vi "Main.vi"() -> ()   [LabVIEW 2023, in "VeriStand Console.lvlib"]
uses:
  VeriStand Console.lvlib
  Message.ctl
  SM Data.ctl
  <vilib>/net/SSH/Client/OpenSSH/OpenSSH Client.lvclass
  Message Queue.ctl
  Login Info.ctl
  <vilib>/net/SSH/NI_SSH.lvlib
panel:
  in  "Disconnect":bool
  out "Connected?":bool
  in  "Connect":bool
  in  "Password":string
  in  "Username":string
  in  "Target Address":string
  in  "Stop":bool
  in  "UI Settings":bool
  out "Console":string
  out "return code":i32
  out "standard error":string
  out "SM Debug Data":T1
  out "elements":T2[](array[typedef])
  out "# elements in queue":i32
  out "Poll rate (s)":dbl
  # "Debug"
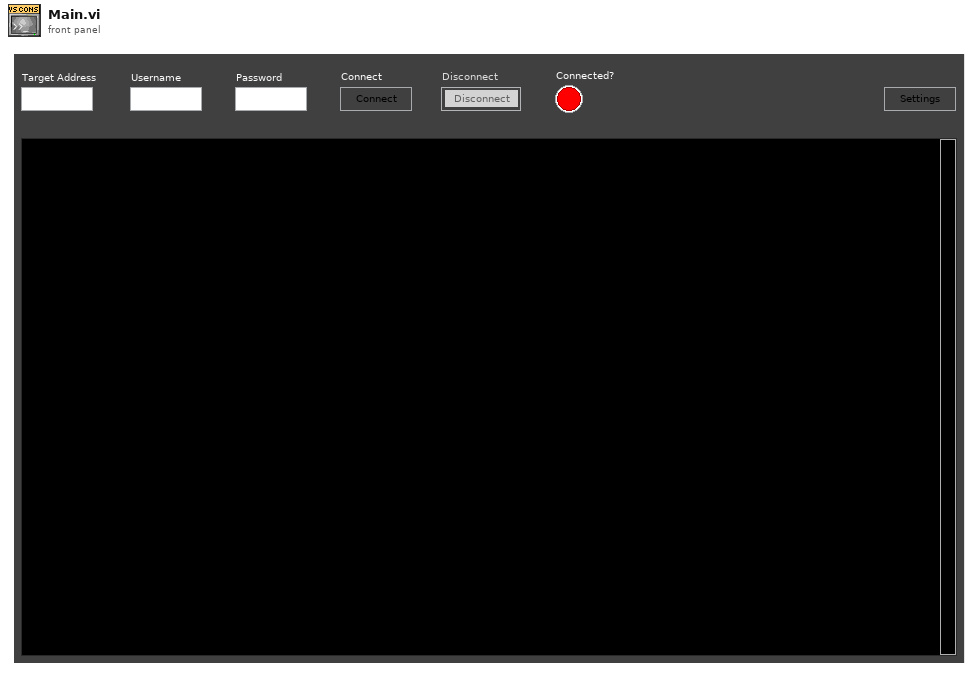
[diagram p1: front panel]
types:
  T1 = typedef "VeriStand Console.lvlib/SM Data.ctl" = cluster{"Connected?":bool, "User@host":string, "NI_SSH.lvlib:OpenSSH Client":refnum<class "OpenSSH Client.lvclass">, "Log file name":string, "Current text":string, "Scroll To Bottom?":bool}
  T2 = typedef "VeriStand Console.lvlib/Message.ctl" = cluster{"Message":string, "Message Data":variant}
  T3 = typedef "VeriStand Console.lvlib/Message Queue.ctl" = refnum<queue>
  T4 = enum8{"Enabled", "Disabled", "Disabled and Grayed Out"}
  T5 = typedef "VeriStand Console.lvlib/Login Info.ctl" = cluster{"Target IP Address":string, "Username":string, "Password":string, "Flush?":bool}
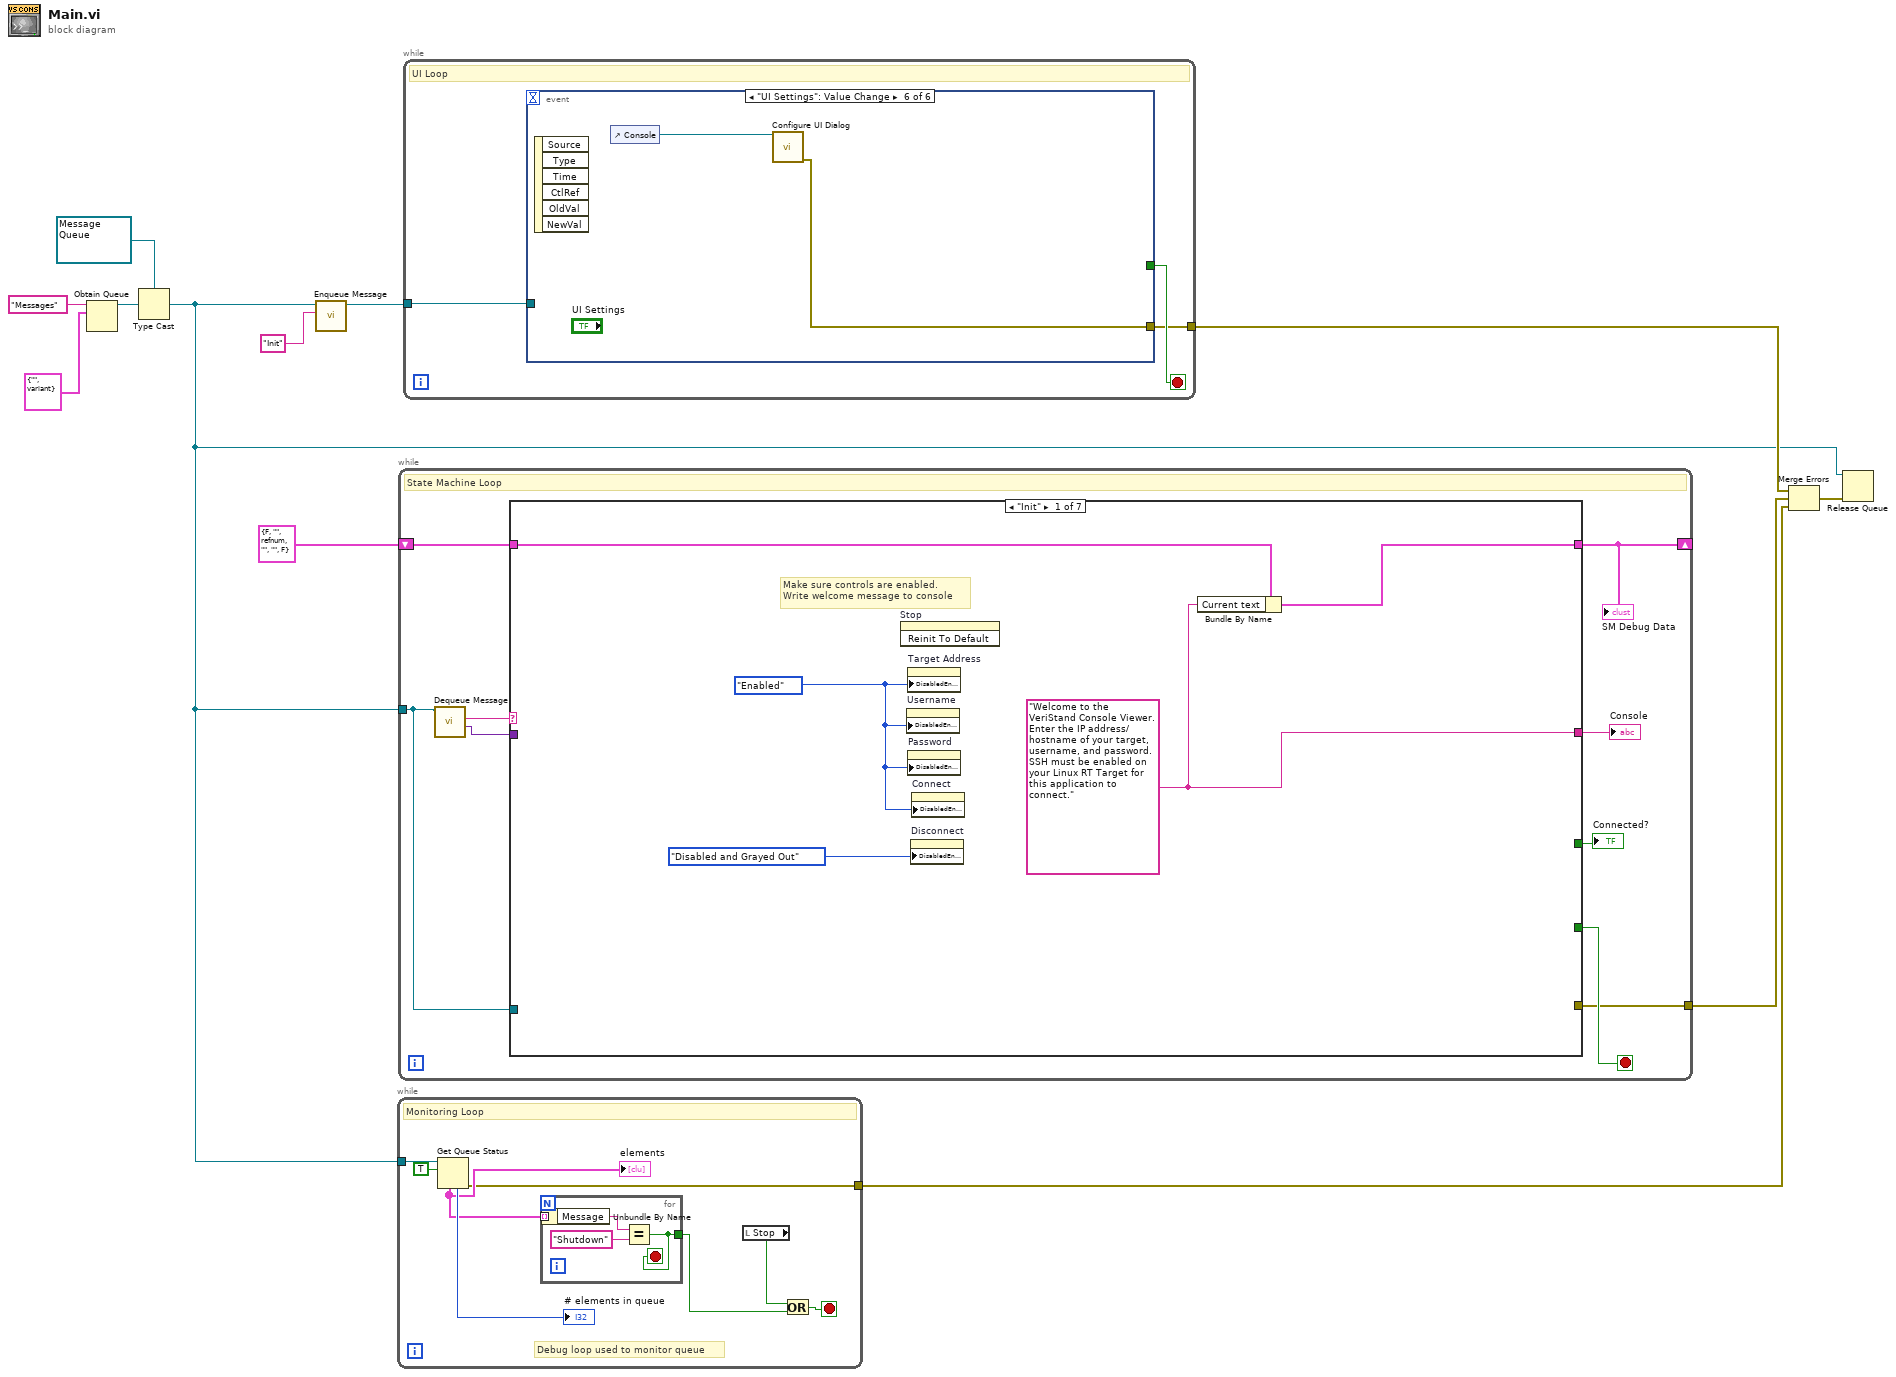
[diagram p0: block diagram]
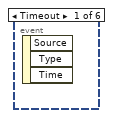
[diagram p2: hidden frame]
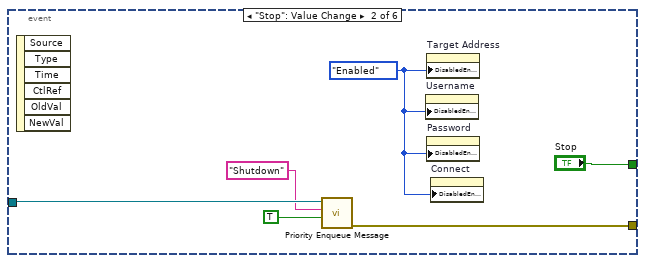
[diagram p3: hidden frame]
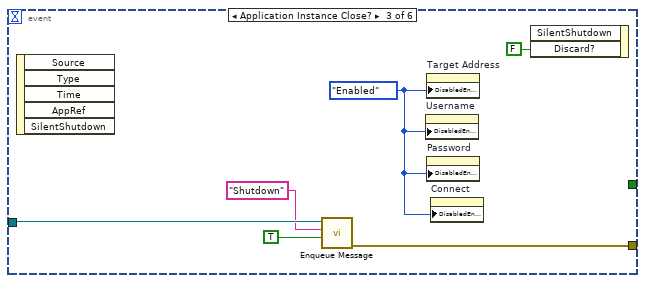
[diagram p4: hidden frame]
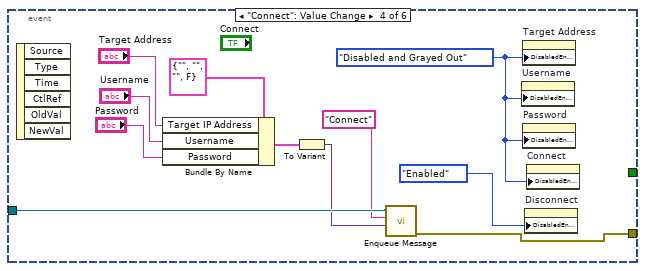
[diagram p5: hidden frame]
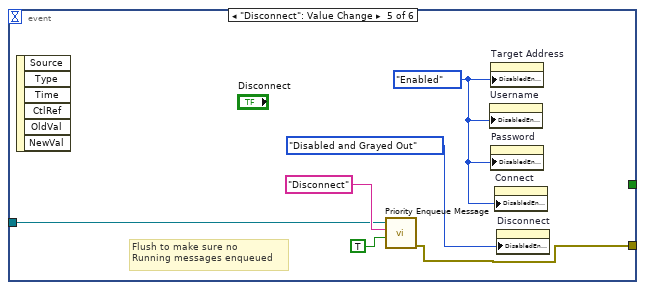
[diagram p6: hidden frame]
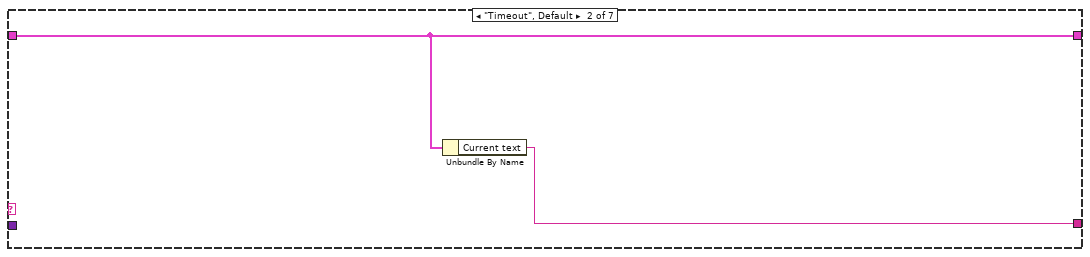
[diagram p7: hidden frame]
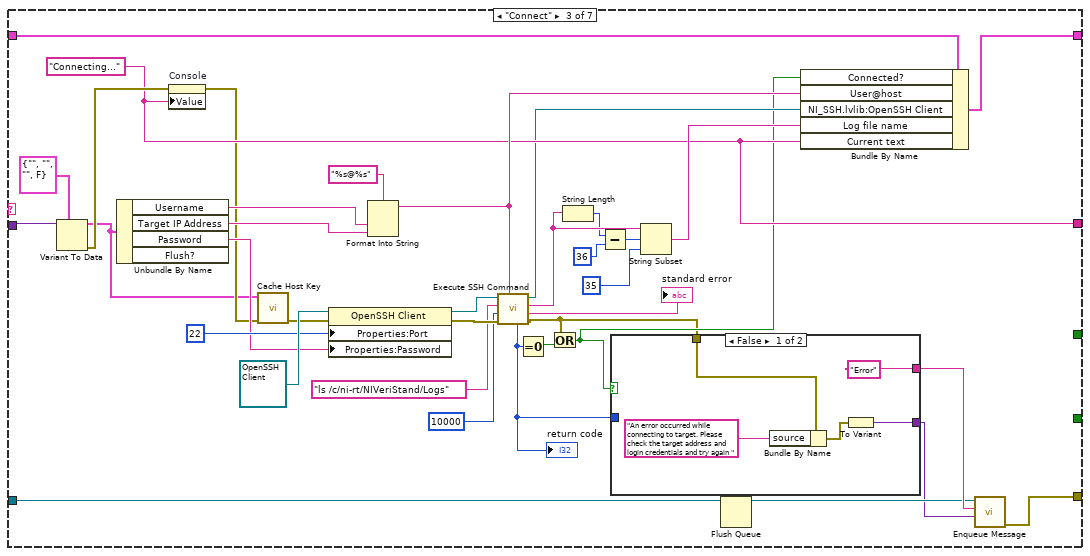
[diagram p8: hidden frame]
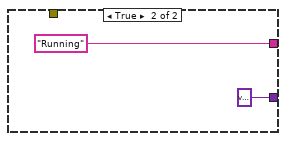
[diagram p9: hidden frame]
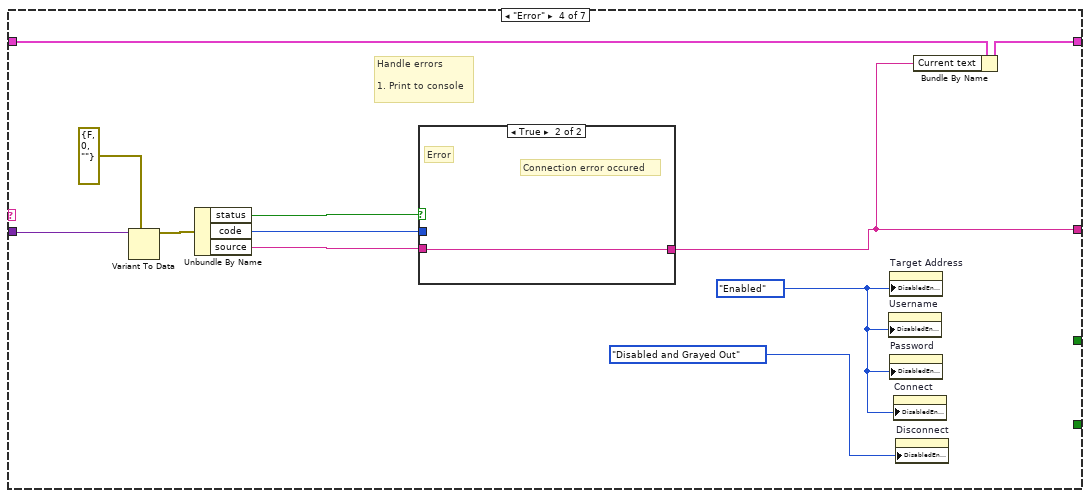
[diagram p10: hidden frame]
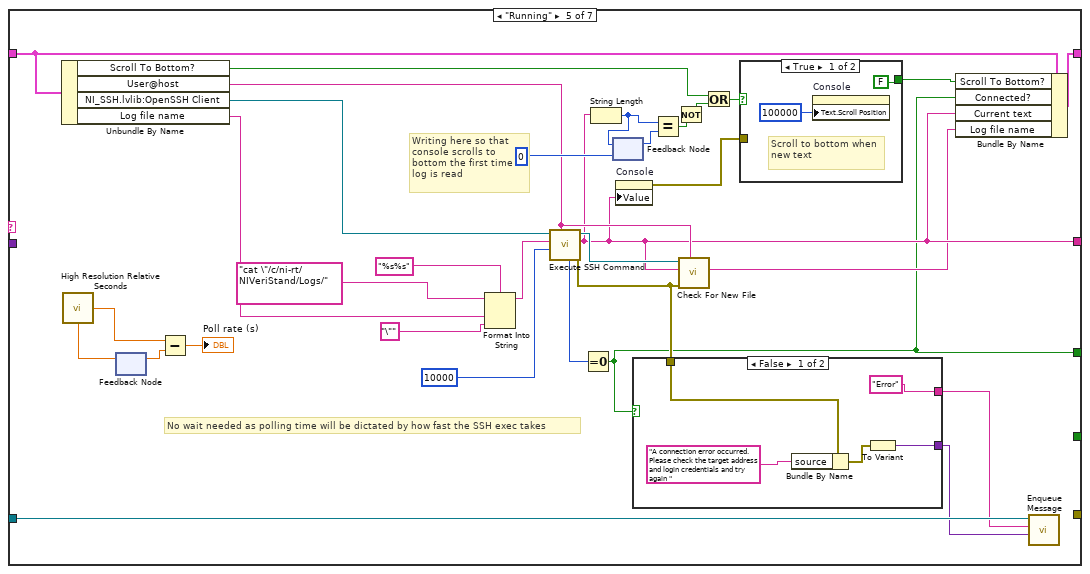
[diagram p12: hidden frame]
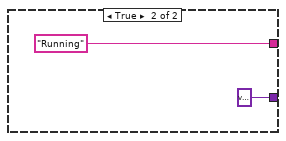
[diagram p13: hidden frame]
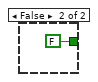
[diagram p14: hidden frame]
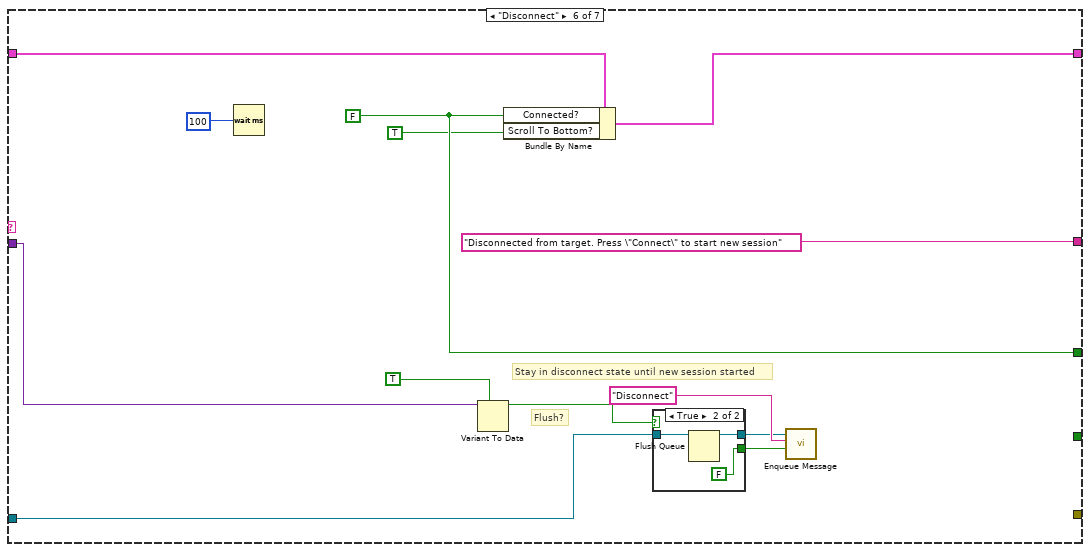
[diagram p15: hidden frame]
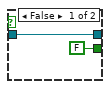
[diagram p16: hidden frame]
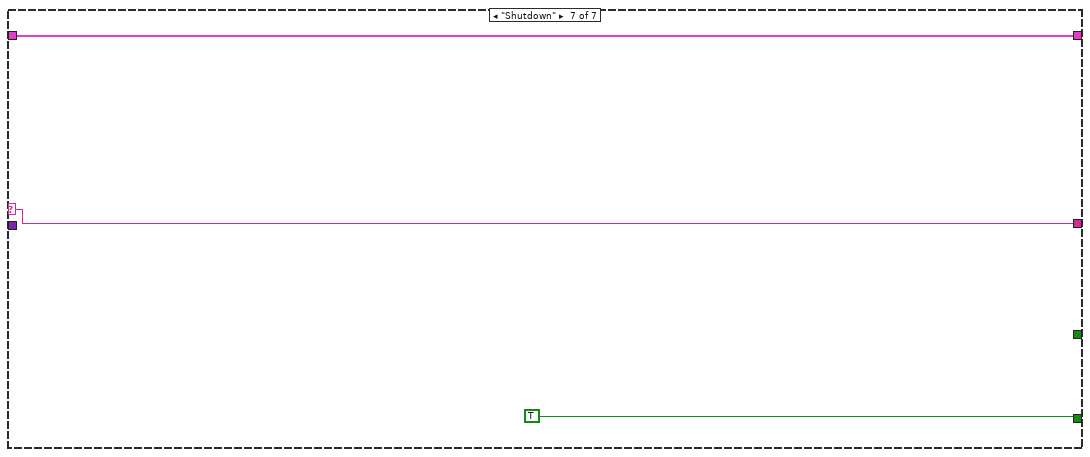
[diagram p17: hidden frame]
diagram:
  n1 = Obtain Queue(name (unnamed)="Messages", element data type=T2 {"Message"="", "Message Data"=variant} ("Message")) -> (queue out=w10:refnum<queue>)  [unwired: 3 in, 2 out]
  n2 = Type Cast(type=T3 refnum ("queue out"), x=w10) -> (*(type *) &x=w1:T3)
  n3 = call "Enqueue Message.vi"("Queue In"=w1, "Message"="Init") -> ("Queue Out"=w6:T3)  [unwired: 6 in, 1 out]
  n4 = while {
    tunnel: w1 -> [w20]
    tunnel: [w16] -> w4
    stop <- w15 stop-if-true
    # "Debug loop used to monitor queue"
    # "Monitoring Loop"
    n5 = Get Queue Status(queue=w20, return elements? (F)=TRUE) -> (error out=w16:errorcluster, # elements in queue=→"# elements in queue":i32, elements=w18:T2[])  [unwired: 1 in, 5 out]
    "elements" <- w18
    n6 = for {
      tunnel: w18 -> [w24] mode=indexing
      tunnel: [w21] -> w14
      stop <- w21 stop-if-true
      n7 = Unbundle By Name(w24) -> ("Message"=w23:string)
      n8 = Equal?(x=w23, y="Shutdown") -> (x = y?=w21:bool)
    }
    n9 = local read "Stop"() -> (w13:bool)
    n10 = Or(x=w13, y=w14) -> (x .or. y?=w15:bool)
  }
  n11 = while {
    tunnel: w1 -> [w26]
    shift-right: [w27] -> _
    shift-left: T1 {"Connected?"=FALSE, "User@host"="", "NI_SSH.lvlib:OpenSSH Client"=refnum, "Log file name"="", "Current text"="", "Scroll To Bottom?"=FALSE} ("SM Data") -> [w28]
    tunnel: [w25] -> w3
    stop <- w33 stop-if-true
    # "State Machine Loop"
    n12 = call "Dequeue Message.vi"("Queue In"=w26) -> ("Message Data"=w31:variant, "Message"=w32:string)  [unwired: 6 in, 3 out]
    n13 = case shown="\"Init\"" w32 {
      selector: w32 -> [_ _ _ _ _ _ w158]
      tunnel: [w35 w40 w52 w87 w104 "Disconnected from target. Press \"Connect\" to start new session" ("standard output") w158] -> w30
      tunnel: [_ _ _ _ _ _ TRUE] -> w33
      tunnel: w31 -> [_ _ w77 w94 _ w143 _]
      tunnel: [_ _ _ _ w98 w148 _] -> w29
      tunnel: w28 -> [w37 w39 w64 w95 w110 w151 w157]
      tunnel: [w36 w39 w63 w88 w109 w150 w157] -> w27
      tunnel: w26 -> [_ _ w55 _ w122 w144 _]
      tunnel: [_ _ w54 _ _ _ _] -> w25
      frame "Init" {
        w38 = T4."Enabled" ("Disabled")
        w35 = "Welcome to the VeriStand Console Viewer. Enter the IP address/hostname of your target, username, and password. SSH must be enabled on your Linux RT Target for this application to connect." ("standard output")
        # "Make sure controls are enabled. \nWrite welcome message to console"
        n14 = invoke on="Stop" class="Bool (strict)" method="Reinit To Default"() -> ()  [unwired: 3 in, 3 out]
        n15 = property on="Username" class="Str"("DisabledEnum"=w38) -> ()  [unwired: 2 in, 2 out]
        n16 = property on="Target Address" class="Str"("DisabledEnum"=w38) -> ()  [unwired: 2 in, 2 out]
        n17 = property on="Password" class="Str"("DisabledEnum"=w38) -> ()  [unwired: 2 in, 2 out]
        n18 = property on="Disconnect" class="Bool"("DisabledEnum"=T4."Disabled and Grayed Out" ("Disabled")) -> ()  [unwired: 2 in, 2 out]
        n19 = property on="Connect" class="Bool"("DisabledEnum"=w38) -> ()  [unwired: 2 in, 2 out]
        n20 = Bundle By Name(cluster=w37, "Current text"=w35) -> (w36:T1)
      }
      frame "Timeout", Default {
        n21 = Unbundle By Name(w39) -> ("Current text"=w40:string)
      }
      frame "Connect" {
        w52 = "Connecting..." ("standard output")
        n22 = Variant To Data(type=T5 {"Target IP Address"="", "Username"="", "Password"="", "Flush?"=FALSE} ("Login Info"), Variant=w77) -> (data=w44:T5, error out=w53:errorcluster)  [unwired: 1 in]
        n23 = Unbundle By Name(w44) -> ("Username"=w71:string, "Target IP Address"=w70:string, "Password"=w68:string)  [unwired: 1 out]
        n24 = property on="Console" class="Str"(error in=w53, "Value"=w52) -> (error out=w45:errorcluster)  [unwired: 1 in, 1 out]
        n25 = call "Cache Host Key.vi"("error in (no error)"=w45, "Login Info"=w44) -> ("error out"=w46:errorcluster)  [unwired: 9 in]
        n26 = property class="OpenSSH Client"(reference=refnum<class "OpenSSH Client.lvclass"> refnum ("NI_SSH.lvlib:OpenSSH Client"), error in=w46, "Properties:Port"=u16 22 ("Port"), "Properties:Password"=w68) -> (reference out=w74:refnum<class "OpenSSH Client.lvclass">, error out=w73:errorcluster)
        n27 = Format Into String(format string="%s@%s", w71, w70) -> (resulting string=w66:string)  [unwired: 2 in, 1 out]
        n28 = call <vilib>:"Execute SSH Command.vi"("user@host"=w66, "error in (no error)"=w73, "timeout (ms)"=10000, "command line"="ls /c/ni-rt/NIVeriStand/Logs", "session in"=w74) -> ("error out"=w41:errorcluster, "standard error"=→"standard error":string, "standard output"=w62:string, "session out"=w48:refnum<class "OpenSSH Client.lvclass">, "return code"=w49:i32)  [unwired: 2 in]
        "return code" <- w49
        n29 = Equal To 0?(x=w49) -> (x = 0?=w42:bool)
        n30 = Or(x=w41, y=w42) -> (x .or. y?=w43:bool)
        n31 = String Length(string=w62) -> (length=w60:i32)
        n32 = Subtract(x=w60, y=36) -> (x-y=w61:i32)
        n33 = case shown="False" w43 {
          tunnel: ["Error" ("Message") "Running" ("Message")] -> w65
          tunnel: [w80 variant ("Variant")] -> w51
          tunnel: w49 -> [_ _]
          tunnel: w41 -> [w78 _]
          frame False {
            n34 = Bundle By Name(cluster=w78, "source"="An error occurred while connecting to target. Please check the target address and login credentials and try again " ("Message")) -> (w81:errorcluster)
            n35 = To Variant(anything=w81) -> (Variant=w80:variant)
          }
          frame True {
          }
        }
        n36 = String Subset(string=w62, offset (0)=w61, length (rest)=35 ("length (rest)")) -> (substring=w58:string)
        n37 = Flush Queue(queue=w55) -> (queue out=w56:T3)  [unwired: 1 in, 2 out]
        n38 = Bundle By Name(cluster=w64, "Connected?"=w43, "User@host"=w66, "NI_SSH.lvlib:OpenSSH Client"=w48, "Log file name"=w58, "Current text"=w52) -> (w63:T1)
        n39 = call "Enqueue Message.vi"("Queue In"=w56, "Message"=w65, "Message Data"=w51) -> ("error out"=w54:errorcluster)  [unwired: 5 in, 1 out]
      }
      frame "Error" {
        w85 = T4."Enabled" ("Disabled")
        # "Handle errors\n\n1. Print to console"
        n40 = Variant To Data(type=errorcluster {"status"=FALSE, "code"=0, "source"=""} ("error in (no error)"), Variant=w94) -> (data=w92:errorcluster)  [unwired: 1 in, 1 out]
        n41 = Unbundle By Name(w92) -> ("status"=w91:bool, "code"=w90:i32, "source"=w89:string)
        n42 = case shown="True" w91 {
          tunnel: w90 -> [_ _]
          tunnel: w89 -> [w96 w97]
          tunnel: [w96 w97] -> w87
          frame False {
            # "Warning"
          }
          frame True {
            # "Connection error occured"
            # "Error"
          }
        }
        n43 = property on="Username" class="Str"("DisabledEnum"=w85) -> ()  [unwired: 2 in, 2 out]
        n44 = property on="Target Address" class="Str"("DisabledEnum"=w85) -> ()  [unwired: 2 in, 2 out]
        n45 = property on="Password" class="Str"("DisabledEnum"=w85) -> ()  [unwired: 2 in, 2 out]
        n46 = property on="Connect" class="Bool"("DisabledEnum"=w85) -> ()  [unwired: 2 in, 2 out]
        n47 = property on="Disconnect" class="Bool"("DisabledEnum"=T4."Disabled and Grayed Out" ("Disabled")) -> ()  [unwired: 2 in, 2 out]
        n48 = Bundle By Name(cluster=w95, "Current text"=w87) -> (w88:T1)
      }
      frame "Running" {
        # "Writing here so that console scrolls to bottom the first time log is read"
        # "No wait needed as polling time will be dictated by how fast the SSH exec takes"
        n49 = Unbundle By Name(w110) -> ("Scroll To Bottom?"=w112:bool, "User@host"=w105:string, "NI_SSH.lvlib:OpenSSH Client"=w123:refnum<class "OpenSSH Client.lvclass">, "Log file name"=w124:string)
        n50 = call <vilib>:"High Resolution Relative Seconds.vi"() -> ("relative seconds"=w116:dbl)
        n51 = feedback-in #1(w116) -> ()
        n52 = feedback #1() -> (w117:dbl)  [unwired: 1 in]
        n53 = Subtract(x=w116, y=w117) -> (x-y=→"Poll rate (s)":dbl)
        n54 = Format Into String(format string="%s%s", initial string="cat \"/c/ni-rt/NIVeriStand/Logs/", w124, "\"" ("input 2")) -> (resulting string=w128:string)  [unwired: 1 in, 1 out]
        n55 = call <vilib>:"Execute SSH Command.vi"("user@host"=w105, "timeout (ms)"=10000, "command line"=w128, "session in"=w123) -> ("error out"=w99:errorcluster, "standard output"=w104:string, "session out"=w106:refnum<class "OpenSSH Client.lvclass">, "return code"=w121:i32)  [unwired: 3 in, 1 out]
        n56 = Equal To 0?(x=w121) -> (x = 0?=w98:bool)
        n57 = String Length(string=w104) -> (length=w120:i32)
        n58 = feedback-in #2(w120) -> ()
        n59 = feedback #2(0) -> (w119:i32)
        n60 = property on="Console" class="Str"("Value"=w104) -> (error out=w114:errorcluster)  [unwired: 2 in, 1 out]
        n61 = case shown="False" w98 {
          tunnel: ["Error" ("Message") "Running" ("Message")] -> w101
          tunnel: [w131 variant ("Variant")] -> w100
          tunnel: w99 -> [w129 _]
          frame False {
            n62 = Bundle By Name(cluster=w129, "source"="A connection error occurred. Please check the target address and login credentials and try again " ("Message")) -> (w132:errorcluster)
            n63 = To Variant(anything=w132) -> (Variant=w131:variant)
          }
          frame True {
          }
        }
        n64 = Equal?(x=w120, y=w119) -> (x = y?=w113:bool)
        n65 = Not(x=w113) -> (.not. x?=w107:bool)
        n66 = call "Check For New File.vi"("user@host"=w105, "error in (no error)"=w99, "Previous file name"=w104, "OpenSSH Client in"=w106) -> ("Next file name"=w103:string)  [unwired: 6 in, 1 out]
        n67 = Or(x=w112, y=w107) -> (x .or. y?=w111:bool)
        n68 = case shown="True" w111 {
          tunnel: w114 -> [_ _]
          tunnel: [FALSE FALSE] -> w108
          frame True {
            # "Scroll to bottom when new text"
            n69 = property on="Console" class="Str"("Text.Scroll Position"=u32 100000) -> ()  [unwired: 2 in, 2 out]
          }
          frame False {
          }
        }
        n70 = Bundle By Name(cluster=w110, "Scroll To Bottom?"=w108, "Connected?"=w98, "Current text"=w104, "Log file name"=w103) -> (w109:T1)
        n71 = call "Enqueue Message.vi"("Queue In"=w122, "Message"=w101, "Message Data"=w100) -> ()  [unwired: 5 in, 2 out]
      }
      frame "Disconnect" {
        w148 = FALSE ("Connected?")
        # "Flush?"
        # "Stay in disconnect state until new session started"
        n72 = Wait (ms)(milliseconds to wait=u32 100) -> ()  [unwired: 1 out]
        n73 = Variant To Data(type=TRUE, Variant=w143) -> (data=w141:bool)  [unwired: 1 in, 1 out]
        n74 = Bundle By Name(cluster=w151, "Connected?"=w148, "Scroll To Bottom?"=TRUE) -> (w150:T1)
        n75 = case shown="True" w141 {
          tunnel: [w153 w156] -> w145
          tunnel: w144 -> [w153 w155]
          tunnel: [FALSE FALSE] -> w140
          frame False {
          }
          frame True {
            n76 = Flush Queue(queue=w155) -> (queue out=w156:T3)  [unwired: 1 in, 2 out]
          }
        }
        n77 = call "Enqueue Message.vi"("Queue In"=w145, "Message"="Disconnect", "Message Data"=w140) -> ()  [unwired: 5 in, 2 out]
      }
      frame "Shutdown" {
      }
    }
    "Console" <- w30
    "Connected?" <- w29
    "SM Debug Data" <- w27
  }
  n78 = while {
    tunnel: w6 -> [w161]
    tunnel: [w160] -> w2
    stop <- w162 stop-if-true
    # "UI Loop"
    n79 = event shown="[5] \"UI Settings\": Value Change" {
      selector: _ -> [_ _ _ _ _ _]
      dyn-events: _ -> [_ _ _ _ _ _]
      timeout: _ -> [_ _ _ _ _ _]
      tunnel: [_ "Stop" _ _ _ _] -> w162
      tunnel: w161 -> [_ w167 w174 w181 w189 _]
      tunnel: [_ w163 w169 w175 w186 w192] -> w160
      event Timeout {
        n80 = event-data() -> ()  [unwired: 1 in, 3 out]
      }
      event "Stop": Value Change {
        w164 = T4."Enabled" ("Disabled")
        n81 = event-data() -> ()  [unwired: 1 in, 6 out]
        n82 = call "Priority Enqueue Message.vi"("Queue In"=w167, "Message"="Shutdown", "Message Data"=TRUE) -> ("error out"=w163:errorcluster)  [unwired: 5 in, 1 out]
        n83 = property on="Username" class="Str"("DisabledEnum"=w164) -> ()  [unwired: 2 in, 2 out]
        n84 = property on="Target Address" class="Str"("DisabledEnum"=w164) -> ()  [unwired: 2 in, 2 out]
        n85 = property on="Password" class="Str"("DisabledEnum"=w164) -> ()  [unwired: 2 in, 2 out]
        n86 = property on="Connect" class="Bool"("DisabledEnum"=w164) -> ()  [unwired: 2 in, 2 out]
      }
      event Application Instance Close? {
        w171 = T4."Enabled" ("Disabled")
        n87 = event-data() -> ()  [unwired: 1 in, 5 out]
        n88 = call "Enqueue Message.vi"("Queue In"=w174, "Message"="Shutdown", "Message Data"=TRUE) -> ("error out"=w169:errorcluster)  [unwired: 5 in, 1 out]
        n89 = property on="Username" class="Str"("DisabledEnum"=w171) -> ()  [unwired: 2 in, 2 out]
        n90 = property on="Target Address" class="Str"("DisabledEnum"=w171) -> ()  [unwired: 2 in, 2 out]
        n91 = property on="Password" class="Str"("DisabledEnum"=w171) -> ()  [unwired: 2 in, 2 out]
        n92 = property on="Connect" class="Bool"("DisabledEnum"=w171) -> ()  [unwired: 2 in, 2 out]
        n93 = event-data("Discard?"=FALSE) -> ()  [unwired: 2 in, 1 out]
      }
      event "Connect": Value Change {
        w177 = T4."Disabled and Grayed Out" ("Disabled")
        n94 = event-data() -> ()  [unwired: 1 in, 6 out]
        n95 = Bundle By Name(cluster=T5 {"Target IP Address"="", "Username"="", "Password"="", "Flush?"=FALSE} ("Login Info"), "Target IP Address"="Target Address", "Username"="Username", "Password"="Password") -> (w180:T5)
        n96 = To Variant(anything=w180) -> (Variant=w179:variant)
        n97 = call "Enqueue Message.vi"("Queue In"=w181, "Message"="Connect", "Message Data"=w179) -> ("error out"=w175:errorcluster)  [unwired: 5 in, 1 out]
        n98 = property on="Username" class="Str"("DisabledEnum"=w177) -> ()  [unwired: 2 in, 2 out]
        n99 = property on="Target Address" class="Str"("DisabledEnum"=w177) -> ()  [unwired: 2 in, 2 out]
        n100 = property on="Password" class="Str"("DisabledEnum"=w177) -> ()  [unwired: 2 in, 2 out]
        n101 = property on="Disconnect" class="Bool"("DisabledEnum"=T4."Enabled" ("Disabled")) -> ()  [unwired: 2 in, 2 out]
        n102 = property on="Connect" class="Bool"("DisabledEnum"=w177) -> ()  [unwired: 2 in, 2 out]
      }
      event "Disconnect": Value Change {
        w190 = T4."Enabled" ("Disabled")
        # "Flush to make sure no\nRunning messages enqueued"
        n103 = event-data() -> ()  [unwired: 1 in, 6 out]
        n104 = call "Priority Enqueue Message.vi"("Queue In"=w189, "Message"="Disconnect", "Message Data"=TRUE) -> ("error out"=w186:errorcluster)  [unwired: 5 in, 1 out]
        n105 = property on="Username" class="Str"("DisabledEnum"=w190) -> ()  [unwired: 2 in, 2 out]
        n106 = property on="Target Address" class="Str"("DisabledEnum"=w190) -> ()  [unwired: 2 in, 2 out]
        n107 = property on="Password" class="Str"("DisabledEnum"=w190) -> ()  [unwired: 2 in, 2 out]
        n108 = property on="Connect" class="Bool"("DisabledEnum"=w190) -> ()  [unwired: 2 in, 2 out]
        n109 = property on="Disconnect" class="Bool"("DisabledEnum"=T4."Disabled and Grayed Out" ("Disabled")) -> ()  [unwired: 2 in, 2 out]
      }
      event "UI Settings": Value Change {
        n110 = event-data() -> ()  [unwired: 1 in, 6 out]
        n111 = control-ref of="Console"() -> (w193:refnum<vi>)
        n112 = call "Configure UI Dialog.vi"("Str Refnum"=w193) -> ("Error out"=w192:errorcluster)  [unwired: 10 in]
      }
    }
  }
  n113 = Merge Errors(w2, w3, w4) -> (w5:errorcluster)
  n114 = Release Queue(queue=w1, error in (no error)=w5) -> ()  [unwired: 1 in, 3 out]
